vi "NI Bring to Front.vi"(0 "Window Name":string, 11 "error in (no error)":errorcluster) -> (15 "error out":errorcluster)   [LabVIEW 2018]
uses:
  user32.dll
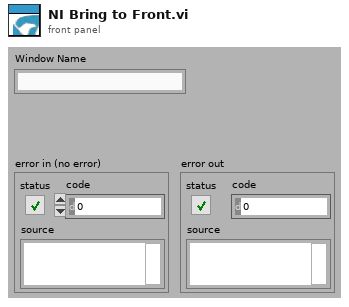
[diagram p1: front panel]
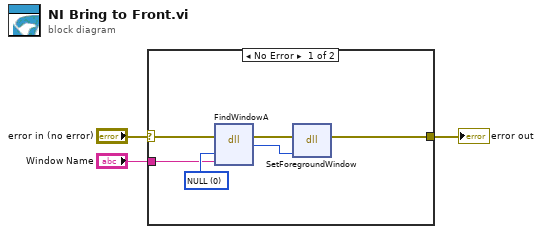
[diagram p0: block diagram]
diagram:
  n1 = case shown="No Error" "error in (no error)" {
    selector: "error in (no error)" -> [w4 w10]
    tunnel: "Window Name" -> [w8 _]
    tunnel: [w5 w10] -> w2
    frame No Error {
      w9 = 0 items=["NULL"]
      n2 = dll-call lib="user32.dll" fn="FindWindowA" label="FindWindow"(error in=w4, "lpszClassName"=w9, "lpszWindowName"=w8) -> (error out=w6:errorcluster, "hWnd"=w7:u32)  [unwired: 3 in, 2 out]
      n3 = dll-call lib="user32.dll" fn="SetForegroundWindow"(error in=w6, "Handle"=w7) -> (error out=w5:errorcluster)  [unwired: 3 in, 2 out]
    }
    frame Error {
    }
  }
  "error out" <- w2
